vi "Get Public API.vi"(8 "error in (no error)":errorcluster, 11 "VoltageUpdate":refnum<class "VoltageUpdate.lvclass">) -> (0 "error out":errorcluster, 2 "Commands":string[](array[string]), 3 "VoltageUpdate out":refnum<class "VoltageUpdate.lvclass">)   [LabVIEW 2016, in "VoltageUpdate.lvclass"]
uses:
  VoltageUpdate.lvclass
  <userlib>/LevyLab/Levylab Instruments/Instrument Types/VSource/Instrument.VSource.lvclass
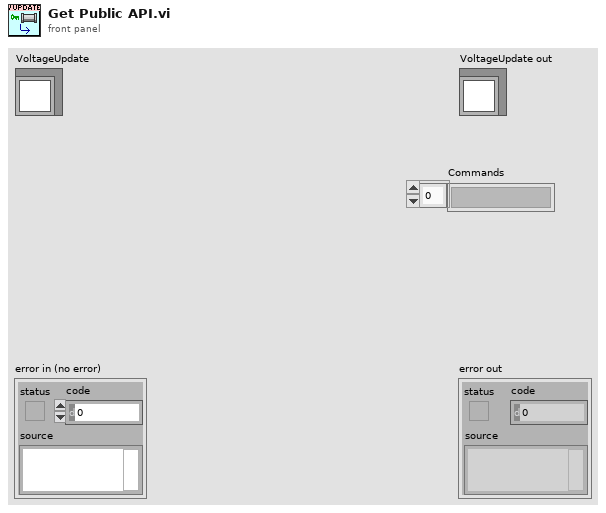
[diagram p1: front panel]
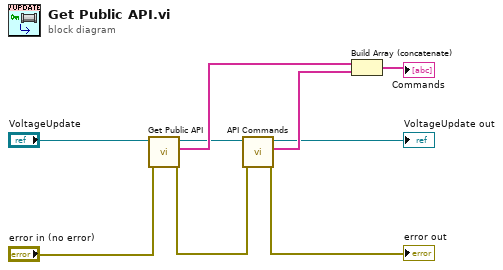
[diagram p0: block diagram]
diagram:
  n1 = call-parent "Get Public API.vi"("error in (no error)"="error in (no error)", "Instrument in"="VoltageUpdate") -> ("error out"=w2:errorcluster, "Commands"=w9:string[], "Instrument out"=w4:refnum<class "VoltageUpdate.lvclass">)  [unwired: 7 in]
  n2 = call "API Commands.vi"("error in (no error)"=w2, "VoltageUpdate in"=w4) -> ("error out"=→"error out":errorcluster, "API Commands"=w5:string[], "VoltageUpdate out"=→"VoltageUpdate out":refnum<class "VoltageUpdate.lvclass">)  [unwired: 7 in]
  n3 = Build Array (concatenate)(w9, w5) -> (→"Commands":string[])
